vi "get handler dataset.vi"(8 "error in":errorcluster, 10 "initial dataset":refnum<class "basic HTTP handler dataset.lvclass">, 11 "TLS HTTP server in":refnum<class "TLS HTTP server.lvclass">) -> (0 "error out":errorcluster, 2 "basic HTTP handler dataset":refnum<class "basic HTTP handler dataset.lvclass">)   [LabVIEW 2016, in "TLS HTTP server.lvclass"]
uses:
  TLS HTTP server.lvclass
  HTTP handler dataset/basic HTTP handler dataset.lvclass
  TLS HTTP server.lvclass/TLS HTTP server.ctl
  TLS handler dataset/TLS HTTP handler dataset.lvclass
  C:/Users/IEUser/Desktop/http/HTTP handler dataset/basic HTTP handler dataset.lvclass
  HTTP server/Basic HTTP server.lvclass
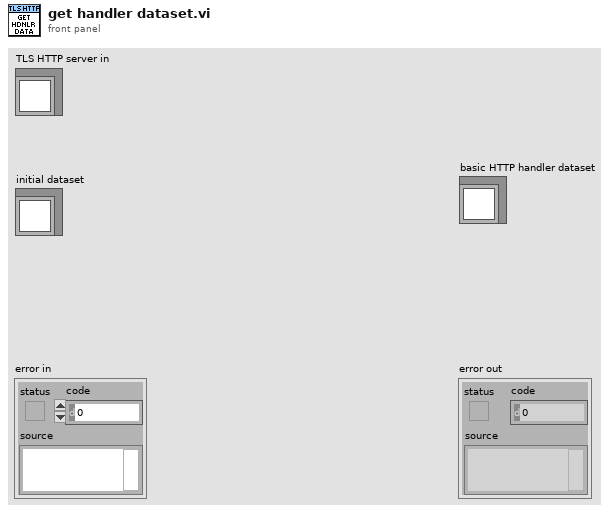
[diagram p1: front panel]
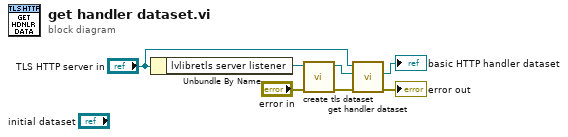
[diagram p0: block diagram]
diagram:
  n1 = Unbundle By Name("TLS HTTP server in") -> ("lvlibretls server listener"=w4:refnum<class "lvlibretls server listener.lvclass">)
  n2 = call "create tls dataset.vi"("error in"="error in", "lvlibretls server listener"=w4) -> ("error out"=w1:errorcluster, "TLS HTTP handler dataset out"=w3:refnum<class "TLS HTTP handler dataset.lvclass">)  [unwired: 8 in]
  n3 = call-parent "get handler dataset.vi"("error in"=w1, "initial dataset"=w3, "Basic HTTP server in"="TLS HTTP server in") -> ("error out"=→"error out":errorcluster, "basic HTTP handler dataset"=→"basic HTTP handler dataset":refnum<class "basic HTTP handler dataset.lvclass">)  [unwired: 7 in]
